vi "Generate_I2C.vi"(8 "Error_In":errorcluster, 10 "Mode":T1, 11 "10Bit_Address_In":refnum<class "10Bit_Address.lvclass">) -> (0 "Error_Out":errorcluster, 3 "10Bit_Address_Out":refnum<class "10Bit_Address.lvclass">)   [LabVIEW 2023, in "10Bit_Address.lvclass"]
uses:
  10Bit_Address.lvclass
  D:/Git/Assignments/SDLC_I2C/SDLC_I2C_LV23V/Class/I2C/I2C.lvclass
  Class/I2C/Controls/Mode.ctl
  Controls/I2C_States.ctl
  10Bit_Address.lvclass/10Bit_Address.ctl
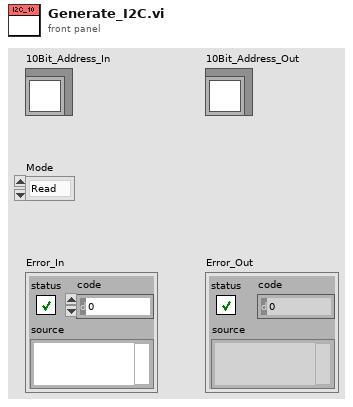
[diagram p1: front panel]
types:
  T1 = typedef "Mode.ctl" = enum16{"Read", "Write"}
  T2 = typedef "I2C_States.ctl" = enum16{"Start", "Byte", "Ack_Nack", "Stop"}
  T3 = typedef "Converted_Data.ctl" = cluster{"Vmin":dbl, "Vmax":dbl, "Input":string, "Off_Set (uS)":dbl, "T_HD_STA (uS)":dbl, "Sample_Per_Us":dbl, "T_HD_DAT (uS)":dbl, "T_SU_DAT (uS)":dbl, "Frequency (kHz)":dbl, "T_SU_STO":dbl, "T_Off (uS)":dbl, "T_On (uS)":dbl, "T_BUF":dbl, "Target_Address":u16, "Register_Address":u8, "Byte_Array":u8[]}
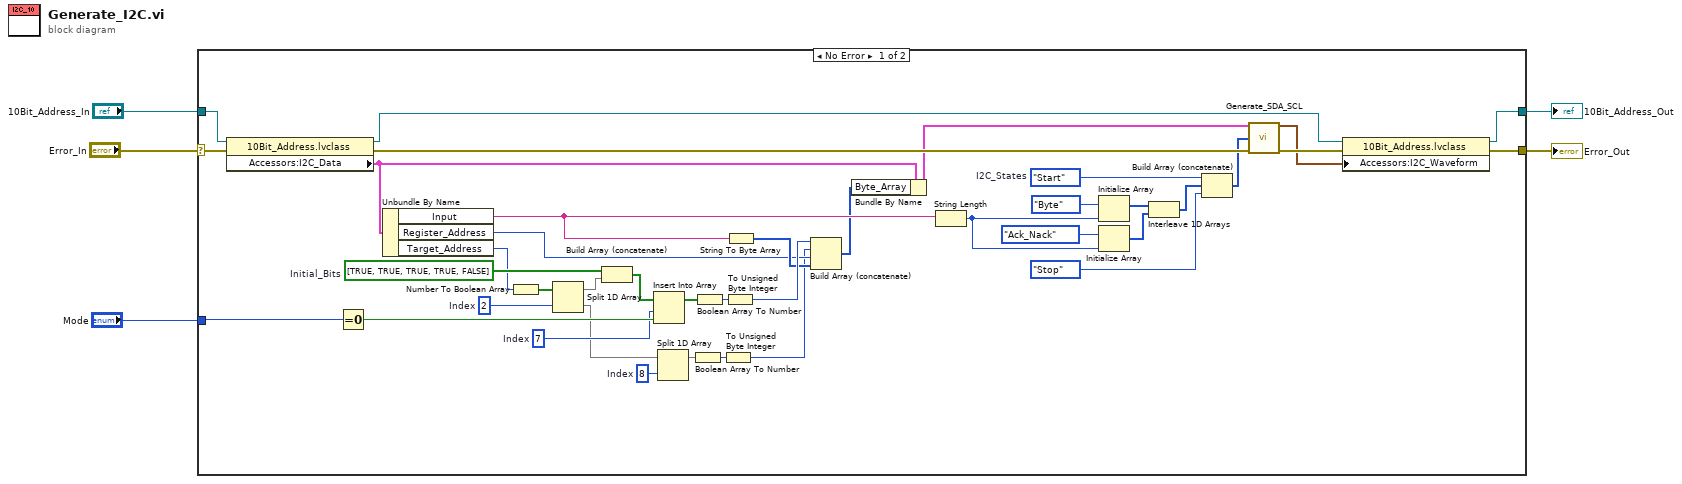
[diagram p0: block diagram]
diagram:
  n1 = case shown="No Error" "Error_In" {
    selector: "Error_In" -> [w44 w47]
    tunnel: [w19 w47] -> w1
    tunnel: [w21 w46] -> w2
    tunnel: "10Bit_Address_In" -> [w33 w46]
    tunnel: "Mode" -> [w29 _]
    frame No Error {
      w10 = 8  # Index
      w16 = bool[] [TRUE, TRUE, TRUE, TRUE, FALSE]  # Initial_Bits
      w17 = 2  # Index
      w27 = 7  # Index
      w42 = I2C_States."Start"  # I2C_States
      n2 = property on="Property Node" class="10Bit_Address.lvclass"(reference=w33, error in=w44) -> (reference out=w32:refnum<class "10Bit_Address.lvclass">, error out=w43:errorcluster, "Accessors:I2C_Data"=w20:T3)
      n3 = Equal To 0?(x=w29) -> (x = 0?=w28:bool)
      n4 = Unbundle By Name(w20) -> ("Input"=w30:string, "Register_Address"=w12:u8, "Target_Address"=w6:u16)
      n5 = Number To Boolean Array(number=w6) -> (Boolean array=w18:bool[])
      n6 = Split 1D Array(array=w18, index=w17) -> (first subarray=w15:bool[], second subarray=w11:bool[])
      n7 = Build Array (concatenate)(w16, w15) -> (w14:bool[])
      n8 = Insert Into Array(array=w14, index=w27, new element=w28) -> (w26:bool[])
      n9 = Split 1D Array(array=w11, index=w10) -> (first subarray=w8:bool[])  [unwired: 1 out]
      n10 = Boolean Array To Number(Boolean array=w8) -> (number=w9:u32)
      n11 = Boolean Array To Number(Boolean array=w26) -> (number=w25:u32)
      n12 = To Unsigned Byte Integer(number=w9) -> (unsigned 8bit integer=w7:u8)
      n13 = To Unsigned Byte Integer(number=w25) -> (unsigned 8bit integer=w24:u8)
      n14 = String To Byte Array(string=w30) -> (unsigned byte array=w13:u8[])
      n15 = Build Array (concatenate)(w24, w7, w12, w13) -> (w22:u8[])
      n16 = Bundle By Name(cluster=w20, "Byte_Array"=w22) -> (w23:T3)
      n17 = String Length(string=w30) -> (length=w40:i32)
      n18 = Initialize Array(I2C_States."Byte" ("Enum"), w40) -> (w38:T2[])
      n19 = Initialize Array(I2C_States."Ack_Nack" ("element"), w40) -> (w37:T2[])
      n20 = Interleave 1D Arrays(w38, w37) -> (w36:T2[])
      n21 = Build Array (concatenate)(w42, w36, I2C_States."Stop" ("element")) -> (w34:T2[])
      n22 = call "Generate_SDA_SCL.vi"("Data"=w23, "Data_Sequence"=w34, "Error_In"=w43) -> ("Waveform Graph"=w31:waveform(dbl)[], "Error_Out"=w45:errorcluster)  [unwired: 11 in]
      n23 = property class="10Bit_Address.lvclass"(reference=w32, error in=w45, "Accessors:I2C_Waveform"=w31) -> (reference out=w21:refnum<class "10Bit_Address.lvclass">, error out=w19:errorcluster)
    }
    frame Error {
    }
  }
  "Error_Out" <- w1
  "10Bit_Address_Out" <- w2
